vi "Add Teams to Map.vi"(11 "Game in":refnum<class "Game.lvclass">) -> (3 "Game out":refnum<class "Game.lvclass">)   [LabVIEW 2020, in "SquareBattle.lvlib" / "Game.lvclass"]
uses:
  Game.lvclass
  Game.lvclass/Game.ctl
  Team/Team.lvclass
  Map/Map.lvclass
  Square/Square.lvclass
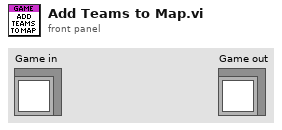
[diagram p1: front panel]
types:
  T1 = typedef "SquareBattle.lvlib/Position.ctl" = cluster{"Row":i32, "Col":i32}
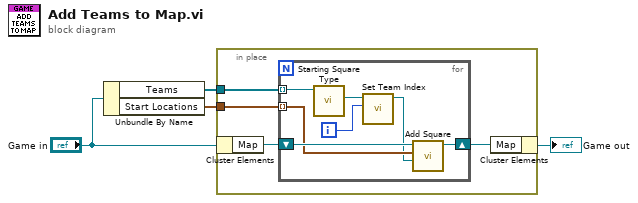
[diagram p0: block diagram]
diagram:
  n1 = Unbundle By Name("Game in") -> ("Teams"=w2:refnum<class "Team.lvclass">[], "Start Locations"=w3:T1[])
  n2 = in-place {
    in-place-border: w3 -> [w6]
    in-place-border: w2 -> [w5]
    n3 = in-place-cluster #1("Game in") -> ("Map"=w8:refnum<class "Map.lvclass">)
    n4 = for {
      shift-right: [w13] -> w7
      shift-left: w8 -> [w15]
      tunnel: w6 -> [w14] mode=indexing
      tunnel: w5 -> [w12] mode=indexing
      i -> [w9]
      n5 = call-dynamic "Starting Square Type.vi"("Team in"=w12) -> ("Square"=w11:refnum<class "Square.lvclass">)  [unwired: 9 in, 1 out]
      n6 = call "Set Team Index.vi"("Team Index"=w9, "Square in"=w11) -> ("Square out"=w10:refnum<class "Square.lvclass">)  [unwired: 8 in, 1 out]
      n7 = call "Add Square.vi"("Square"=w10, "Position"=w14, "Map in"=w15) -> ("Map out"=w13:refnum<class "Map.lvclass">)  [unwired: 7 in, 1 out]
    }
    n8 = in-place-cluster #1("Map"=w7) -> (→"Game out":refnum<class "Game.lvclass">)
  }
